vi "断电保存全局.vi"() -> ()   [LabVIEW 2016]
panel:
  in  "判断数据反馈":bool
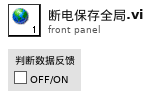
[diagram p1: front panel]
diagram:
